vi "Initialise.vi"(8 "error in (no error)":errorcluster, 10 "Message in":refnum<class "InitialiseMessage.lvclass">, 11 "RSA in":refnum<class "RSA.lvclass">) -> (0 "error out":errorcluster, 3 "RSA out":refnum<class "RSA.lvclass">)   [LabVIEW 2012, in "RSA.lvclass"]
doc: "This method is called when an initialise message is received. It mainly initialises the RabbitMQ connectivity. \n\nOverride this method when your component needs special initialisation (e.g. of software or hardware resources). In that case, don't forget to call the parent for proper implementation. If your component owns subcomponents, they count as resources, so you have to initialise them by calling their own initialise functions"
uses:
  RSA.lvclass
  <vilib>/Distrio/Murmex/InitialiseMessage/InitialiseMessage.lvclass
  <vilib>/Distrio/Murmex/Murmex/Murmex.lvclass
  RSA.lvclass/RSA.ctl
panel:
  # "This method is called when the INTIALISE\ntrigger is sent. \n\nOverride this method when your component needs to\nrespond to this trigger. \n\nCall parent for proper implementation"
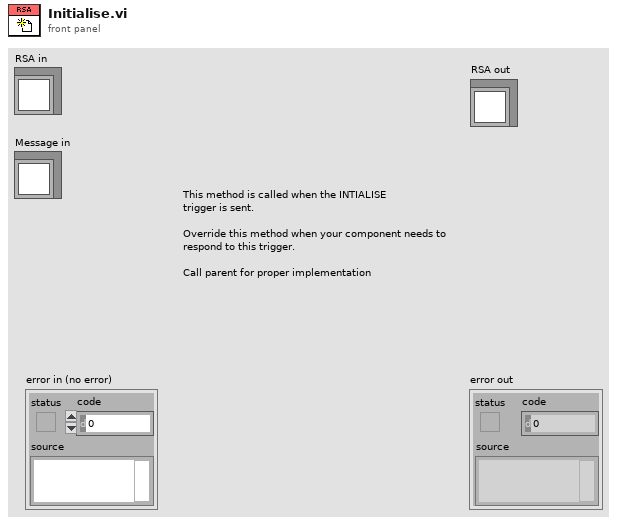
[diagram p1: front panel]
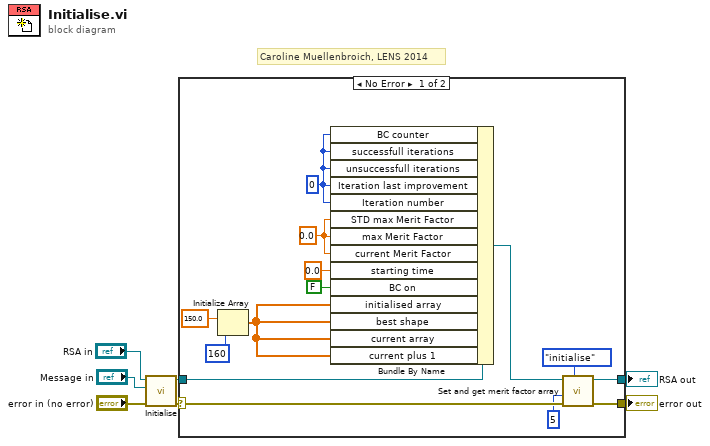
[diagram p0: block diagram]
diagram:
  # "Caroline Muellenbroich, LENS 2014"
  n1 = call-parent "Initialise.vi"("error in (no error)"="error in (no error)", "Message in"="Message in", "Murmex in"="RSA in") -> ("error out"=w4:errorcluster, "Murmex out"=w2:refnum<class "RSA.lvclass">)  [unwired: 7 in]
  n2 = case shown="No Error" w4 {
    selector: w4 -> [w13 w22]
    tunnel: [w12 w22] -> w3
    tunnel: [w10 w23] -> w1
    tunnel: w2 -> [w19 w23]
    frame No Error {
      w17 = 0 ("Run time cluster.Iteration number")
      w18 = 0.0 ("Run time cluster.current Merit Factor")
      n3 = Initialize Array(150.0 ("element"), 160 ("dimension size")) -> (w15:dbl[])
      n4 = Bundle By Name(cluster=w19, "BC counter"=w17, "successfull iterations"=w17, "unsuccessfull iterations"=w17, "Iteration last improvement"=w17, "Iteration number"=w17, "STD max Merit Factor"=w18, "max Merit Factor"=w18, "current Merit Factor"=w18, "starting time"=0.0 ("Run time cluster.starting time"), "BC on"=FALSE ("Run time cluster.Observer ready"), "initialised array"=w15, "best shape"=w15, "current array"=w15, "current plus 1"=w15) -> (w11:refnum<class "RSA.lvclass">)
      n5 = call "Set and get merit factor array.vi"("action"=enum16{"set", "get", "initialise"}."initialise", "error in (no error)"=w13, "array size"=5, "RSA in"=w11) -> ("error out"=w12:errorcluster, "RSA out"=w10:refnum<class "RSA.lvclass">)  [unwired: 4 in, 2 out]
    }
    frame Error {
    }
  }
  "error out" <- w3
  "RSA out" <- w1
